vi "Backpressure - drop notice.vi"(8 "error in (no error)":errorcluster) -> (0 "error out":errorcluster)   [LabVIEW 2026, in "Tests.lvlib"]
doc: "Verifies the synthetic drop-notice record (SRS-LMBR-059): calls BuildDropNotice with sample counts and asserts the rendered message, the protected ERROR level, and the reserved lumberjack.dropped sourceTag.\n\nImplements LMBR-T-051 -> SRS-059. Assert-level IDs: Test-ID-Assert-Checklist.md."
uses:
  Tests.lvlib
  src/TypeDefs/Severity.ctl
  <vilib>/addons/_JKI Toolkits/Caraya/classes/Assert/Assert Equal Value_Variant.vi
  <vilib>/addons/_JKI Toolkits/Caraya/classes/Assert/Assert.lvclass
  <vilib>/addons/_JKI Toolkits/Caraya/classes/Test/Test.lvclass
  src/Lumberjack.lvlib
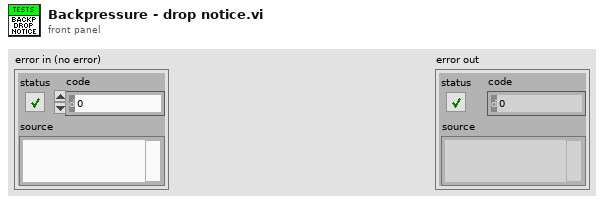
[diagram p1: front panel]
types:
  T1 = typedef "Lumberjack.lvlib/Severity.ctl" = enum16{"OFF", "FATAL", "ERROR", "WARN", "INFO", "DEBUG", "TRACE", "ALL"}
  T2 = typedef "Lumberjack.lvlib/Statement.ctl" = cluster{"timestamp":timestamp, "level":T1, "sourceTag":string, "originVI":string, "message":string}
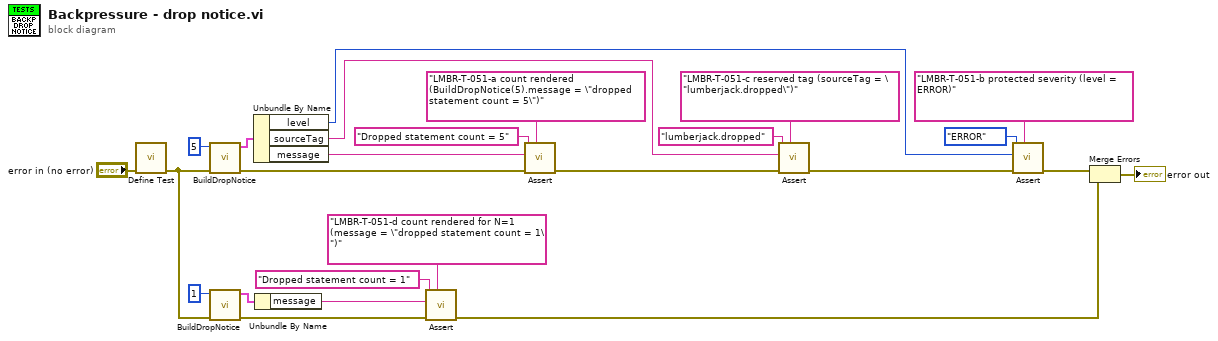
[diagram p0: block diagram]
diagram:
  n1 = call <vilib>:"Define Test.vi"("error in (no error)"="error in (no error)") -> ("error out"=w22:errorcluster)  [unwired: 9 in, 1 out]
  n2 = call "BuildDropNotice.vi"("error in (no error)"=w22, "droppeedCount"=5) -> ("error out"=w18:errorcluster, "Statement"=w19:T2)  [unwired: 8 in]
  n3 = call "BuildDropNotice.vi"("error in (no error)"=w22, "droppeedCount"=1) -> ("error out"=w5:errorcluster, "Statement"=w4:T2)  [unwired: 8 in]
  n4 = Unbundle By Name(w19) -> ("level"=w10:T1, "sourceTag"=w9:string, "message"=w14:string)
  n5 = Unbundle By Name(w4) -> ("message"=w7:string)
  n6 = call-poly <vilib>:"Assert.vi"("Label"="LMBR-T-051-d count rendered for N=1 (message = \"dropped statement count = 1\")" ("sourceTag"), "error in (no error)"=w5, "Actual"=w7, "Expected"="Dropped statement count = 1") -> ("error out"=w3:errorcluster)  [unwired: 6 in, 1 out]
  n7 = call-poly <vilib>:"Assert.vi"("Label"="LMBR-T-051-a count rendered (BuildDropNotice(5).message = \"dropped statement count = 5\")" ("sourceTag"), "error in (no error)"=w18, "Actual"=w14, "Expected"="Dropped statement count = 5") -> ("error out"=w17:errorcluster)  [unwired: 6 in, 1 out]
  n8 = call-poly <vilib>:"Assert.vi"("Label"="LMBR-T-051-c reserved tag (sourceTag = \"lumberjack.dropped\")" ("sourceTag"), "error in (no error)"=w17, "Actual"=w9, "Expected"="lumberjack.dropped") -> ("error out"=w23:errorcluster)  [unwired: 6 in, 1 out]
  n9 = call-poly <vilib>:"Assert.vi"("Label"="LMBR-T-051-b protected severity (level = ERROR)" ("sourceTag"), "error in (no error)"=w23, "Actual"=w10, "Expected"=Severity."ERROR" ("level")) -> ("error out"=w2:errorcluster)  [unwired: 6 in, 1 out]
  n10 = Merge Errors(w2, w3) -> (→"error out":errorcluster)
